vi "gentec-M-Link.Query Head Attributes.vi"(0 "VISA resource In":refnum<visa-resource-name>, 5 "error in (no error)":errorcluster) -> (11 "all Data read":string, 13 "Any Timeout?":bool, 14 "VISA resource Out":refnum<visa-resource-name>, 16 "Head Attributes":T1 {"max. Range" items=["1f", "3f", "10f", "30f", "100f", "300f", "1p", "3p", "10p", "30p", "100p", "300p", "1n", "3n", "10n", "30n", "100n", "300n", "1u", "3u", "10u", "30u", "100u", "300u", "1m", "3m", "10m", "30m", "100m", "300m", "1", "3", "10", "30", "100", "300", "1K", "3K", "10K", "30K", "100K", "300K", "1M", "3M", "10M", "30M", "100M", "300M"]; "Range" items=["1f", "3f", "10f", "30f", "100f", "300f", "1p", "3p", "10p", "30p", "100p", "300p", "1n", "3n", "10n", "30n", "100n", "300n", "1u", "3u", "10u", "30u", "100u", "300u", "1m", "3m", "10m", "30m", "100m", "300m", "1", "3", "10", "30", "100", "300", "1K", "3K", "10K", "30K", "100K", "300K", "1M", "3M", "10M", "30M", "100M", "300M"]}, 19 "error out":errorcluster)   [LabVIEW 2014, in "gentec-M-Link - Driver.lvlib"]
doc: "Data to write: hed"
uses:
  gentec-M-Link - Driver.lvlib
  Type Defs/gentec-M-Link.Head Attributes.ctl
  Type Defs/gentec-M-Link.Range.ctl
panel:
  in  "Head Attributes Dummy":T1 {"max. Range" items=["1f", "3f", "10f", "30f", "100f", "300f", "1p", "3p", "10p", "30p", "100p", "300p", "1n", "3n", "10n", "30n", "100n", "300n", "1u", "3u", "10u", "30u", "100u", "300u", "1m", "3m", "10m", "30m", "100m", "300m", "1", "3", "10", "30", "100", "300", "1K", "3K", "10K", "30K", "100K", "300K", "1M", "3M", "10M", "30M", "100M", "300M"]; "Range" items=["1f", "3f", "10f", "30f", "100f", "300f", "1p", "3p", "10p", "30p", "100p", "300p", "1n", "3n", "10n", "30n", "100n", "300n", "1u", "3u", "10u", "30u", "100u", "300u", "1m", "3m", "10m", "30m", "100m", "300m", "1", "3", "10", "30", "100", "300", "1K", "3K", "10K", "30K", "100K", "300K", "1M", "3M", "10M", "30M", "100M", "300M"]}
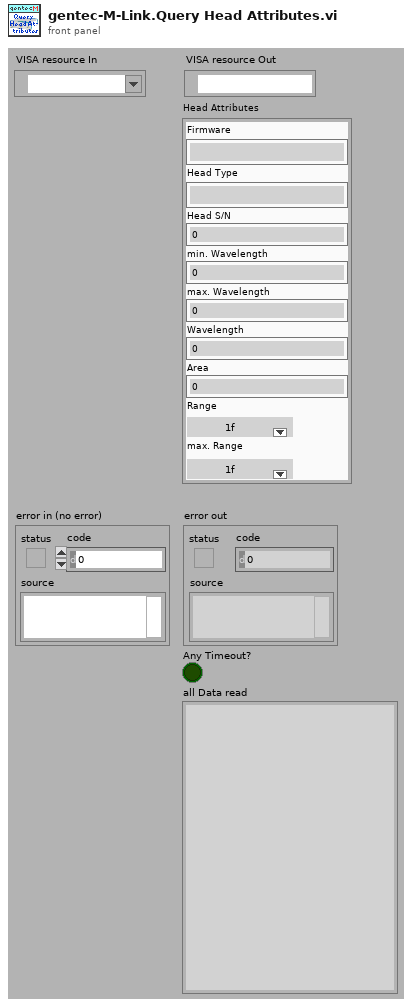
[diagram p1: front panel]
types:
  T1 = typedef "gentec-M-Link - Driver.lvlib/gentec-M-Link.Head Attributes.ctl" = cluster{"Firmware":string, "Head Type":string, "Head S/N":u32, "min. Wavelength":dbl, "max. Wavelength":dbl, "Wavelength":dbl, "Area":dbl, "Range":T2, "max. Range":T2}
  T2 = typedef "gentec-M-Link - Driver.lvlib/gentec-M-Link.Range.ctl" = u16
  T3 = cluster{"[0]":string, "[1]":string, "[2]":string, "[3]":string, "[4]":string, "[5]":string, "[6]":string, "[7]":string, "[8]":string, "[9]":string, "[10]":string, "[11]":string, "[12]":string, "[13]":string}
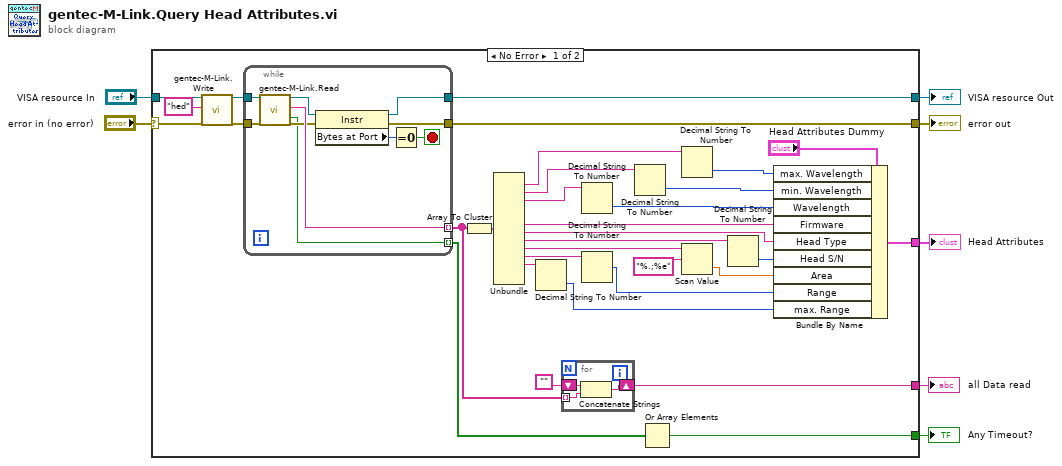
[diagram p0: block diagram]
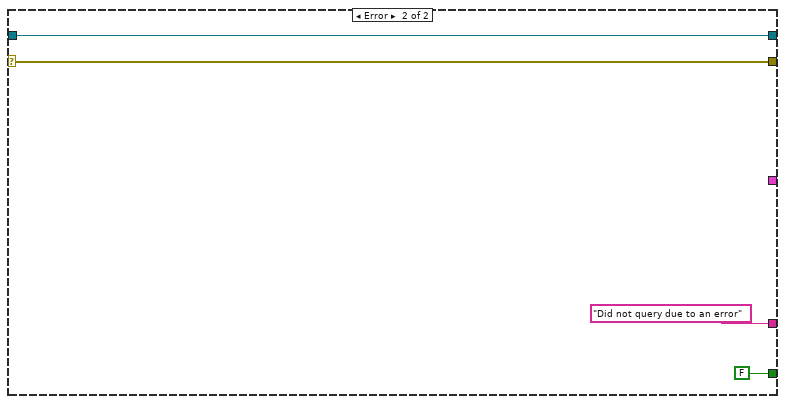
[diagram p2: hidden frame]
diagram:
  n1 = case shown="No Error" "error in (no error)" {
    selector: "error in (no error)" -> [w37 w56]
    tunnel: [w39 w56] -> w6
    tunnel: "VISA resource In" -> [w36 w55]
    tunnel: [w35 w55] -> w4
    tunnel: [w32 _] -> w3
    tunnel: [w11 FALSE] -> w1
    tunnel: [w8 "Did not query due to an error" ("Data Read")] -> w2
    frame No Error {
      n2 = call "gentec-M-Link.Write.vi"("VISA resource (In)"=w36, "Data To Write"="hed", "error in (no error)"=w37) -> ("VISA resource (Out)"=w15:refnum<visa-resource-name>, "error out"=w14:errorcluster)  [unwired: 14 in, 1 out]
      n3 = while {
        tunnel: [w46] -> w39
        tunnel: w15 -> [w52]
        tunnel: w14 -> [w51]
        tunnel: [w50] -> w9 mode=indexing
        tunnel: [w48] -> w35
        tunnel: [w43] -> w12 mode=indexing
        stop <- w44 stop-if-true
        n4 = call "gentec-M-Link.Read.vi"("VISA resource (In)"=w52, "error in (no error)"=w51) -> ("VISA resource (Out)"=w49:refnum<visa-resource-name>, "Data Read"=w50:string, "Read Timeout"=w43:bool, "error out"=w47:errorcluster)  [unwired: 13 in, 1 out]
        n5 = property class="Instr"(reference=w49, error in=w47) -> (reference out=w48:refnum<visa-resource-name>, error out=w46:errorcluster, "Bytes at Port"=w45:u32)
        n6 = Equal To 0?(x=w45) -> (x = 0?=w44:bool)
      }
      n7 = Array To Cluster(array=w9) -> (cluster=w34:T3)
      n8 = Unbundle(w34) -> ("[1]"=w27:string, "[2]"=w25:string, "[3]"=w24:string, "[6]"=w31:string, "[7]"=w30:string, "[8]"=w29:string, "[9]"=w17:string, "[10]"=w21:string, "[11]"=w20:string)  [unwired: 5 out]
      n9 = Decimal String To Number(string=w20) -> (number=w18:i32)  [unwired: 2 in, 1 out]
      n10 = for {
        tunnel: w9 -> [w42] mode=indexing
        shift-right: [w41] -> w8
        shift-left: "" -> [w40]
        n11 = Concatenate Strings(w40, w42) -> (w41:string)
      }
      n12 = Decimal String To Number(string=w24) -> (number=w23:i32)  [unwired: 2 in, 1 out]
      n13 = Decimal String To Number(string=w21) -> (number=w19:i32)  [unwired: 2 in, 1 out]
      n14 = Decimal String To Number(string=w25) -> (number=w22:i32)  [unwired: 2 in, 1 out]
      n15 = Or Array Elements(Boolean array=w12) -> (logical OR=w11:bool)
      n16 = Decimal String To Number(string=w27) -> (number=w26:i32)  [unwired: 2 in, 1 out]
      n17 = Scan Value(string=w17, format string="%.;%e") -> (value=w16:dbl)  [unwired: 1 in, 1 out]
      n18 = Decimal String To Number(string=w29) -> (number=w28:i32)  [unwired: 2 in, 1 out]
      n19 = Bundle By Name(cluster="Head Attributes Dummy", "max. Wavelength"=w26, "min. Wavelength"=w22, "Wavelength"=w23, "Firmware"=w31, "Head Type"=w30, "Head S/N"=w28, "Area"=w16, "Range"=w19, "max. Range"=w18) -> (w32:T1)
    }
    frame Error {
    }
  }
  "error out" <- w6
  "VISA resource Out" <- w4
  "Head Attributes" <- w3
  "all Data read" <- w2
  "Any Timeout?" <- w1
